vi "ArrayView2005.vi"   [LabVIEW 2013]
uses:
  <vilib>/Heliosphere Research LLC/Advanced Plotting Toolkit/Advanced Plotting Toolkit.lvlib
types:
  T1 = typedef "Advanced Plotting Toolkit.lvlib/PlotID.ctl" = i32
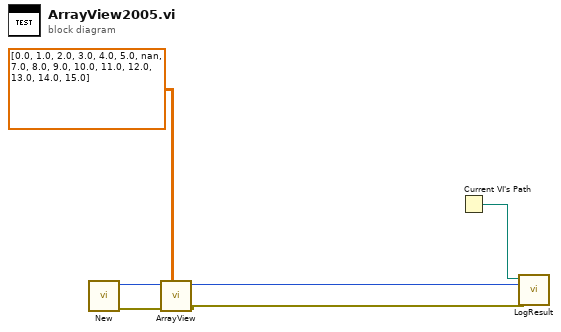
[diagram p0: block diagram]
diagram:
  n1 = call <vilib>:"New.vi"() -> ("error out"=w2:errorcluster, "Plot ID"=w3:T1)  [unwired: 10 in]
  n2 = call <vilib>:"ArrayView.vi"("Data"=dbl[][] [[0.0, 1.0, 2.0, 3.0], [4.0, 5.0, nan, 7.0], [8.0, 9.0, 10.0, 11.0], [12.0, 13.0, 14.0, 15.0]], "error in (no error)"=w2, "Plot ID"=w3) -> ("error out"=w1:errorcluster, "Plot ID Out"=w4:T1)  [unwired: 7 in]
  n3 = Current VI's Path() -> (path=w6:path)
  n4 = call "LogResult.vi"("Test Result"=w1, "Test Artifact"=w4, "VI Path"=w6) -> ()  [unwired: 9 in]
